vi "Fit Radius to Draw Area.vi"(5 "Legend Width":u32, 7 "Title Height":u32, 9 "Selection Popout Offset":i16, 10 "Margin":i16, 11 "Draw Area Size":T1) -> (3 "Radius":i16)   [LabVIEW 2020, in "PieChart.lvclass"]
uses:
  PieChart.lvclass
  <vilib>/Utility/miscctls.llb/LVBoundsTypeDef.ctl
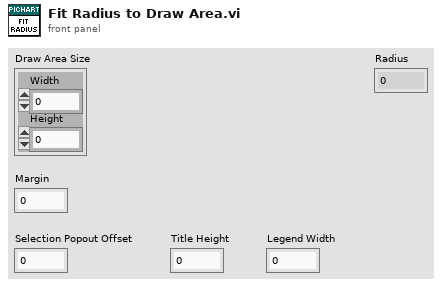
[diagram p1: front panel]
types:
  T1 = typedef "LVBoundsTypeDef.ctl" = cluster{"Width":u32, "Height":u32}
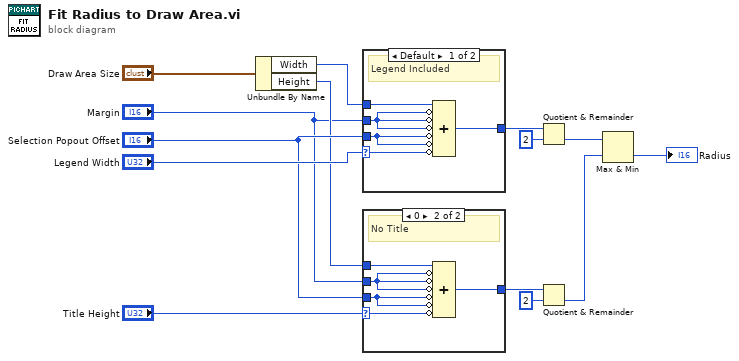
[diagram p0: block diagram]
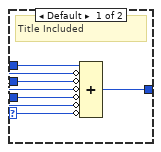
[diagram p2: hidden frame]
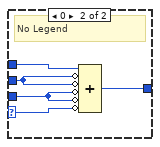
[diagram p3: hidden frame]
diagram:
  n1 = Unbundle By Name("Draw Area Size") -> ("Width"=w3:u32, "Height"=w2:u32)
  n2 = case shown="Default" "Legend Width" {
    selector: "Legend Width" -> [w19 w24]
    tunnel: "Selection Popout Offset" -> [w18 w23]
    tunnel: [w17 w22] -> w6
    tunnel: w3 -> [w16 w21]
    tunnel: "Margin" -> [w15 w20]
    frame Default {
      # "Legend Included"
      n3 = Compound Arithmetic op=ADD(w16, invert w15, invert w15, invert w15, invert w18, invert w18, invert w19) -> (w17:u32)
    }
    frame 0 {
      # "No Legend"
      n4 = Compound Arithmetic op=ADD(w21, invert w20, invert w20, invert w23, invert w23, invert w24) -> (w22:u32)
    }
  }
  n5 = case shown="0" "Title Height" {
    selector: "Title Height" -> [w29 w34]
    tunnel: "Selection Popout Offset" -> [w28 w33]
    tunnel: [w27 w32] -> w10
    tunnel: w2 -> [w26 w31]
    tunnel: "Margin" -> [w25 w30]
    frame Default {
      # "Title Included"
      n6 = Compound Arithmetic op=ADD(w26, invert w25, invert w25, invert w25, invert w28, invert w28, invert w29) -> (w27:u32)
    }
    frame 0 {
      # "No Title"
      n7 = Compound Arithmetic op=ADD(w31, invert w30, invert w30, invert w30, invert w33, invert w33, invert w34) -> (w32:u32)
    }
  }
  n8 = Quotient & Remainder(x=w6, y=u32 2) -> (floor(x/y)=w8:u32)  [unwired: 1 out]
  n9 = Quotient & Remainder(x=w10, y=u32 2) -> (floor(x/y)=w12:u32)  [unwired: 1 out]
  n10 = Max & Min(x=w8, y=w12) -> (min(x,y)=→"Radius":u32)  [unwired: 1 out]
